vi "Init notes.vi"(11 "?":T1={"Tytuły"=[], "Folder"=path "", "Data/tytul"=[], "Ostatni index"=-10, "Title"="", "Note"=""}) -> (3 "?":T1={"Tytuły"=[], "Folder"=path "", "Data/tytul"=[], "Ostatni index"=-10, "Title"="", "Note"=""})   [LabVIEW 2020]
uses:
  #typeDef_ProgramData.ctl
  <vilib>/regexp/Match Regular Expression.xnode
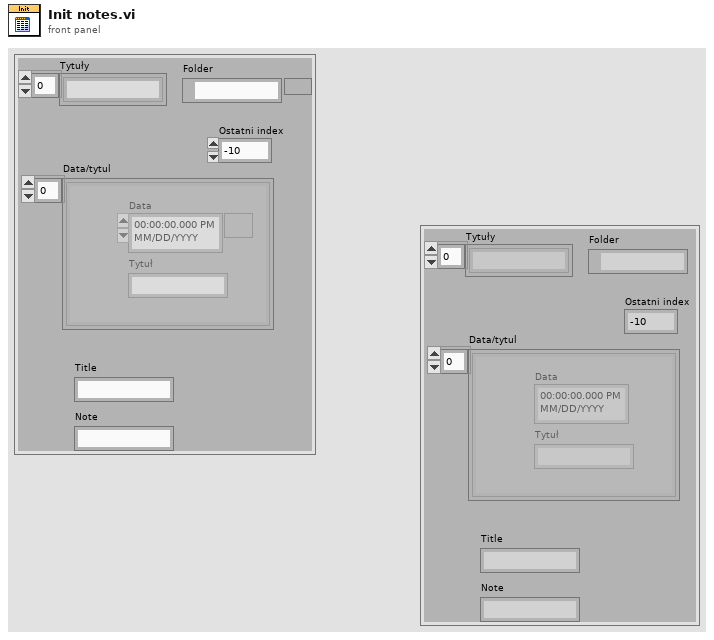
[diagram p1: front panel]
types:
  T1 = typedef "#typeDef_ProgramData.ctl" = cluster{"Tytuły":string[], "Folder":path, "Data/tytul":cluster{"Data":timestamp, "Tytuł":string}[], "Ostatni index":i32, "Title":string, "Note":string}
  T2 = cluster{"last mod":timestamp, "before match":string}
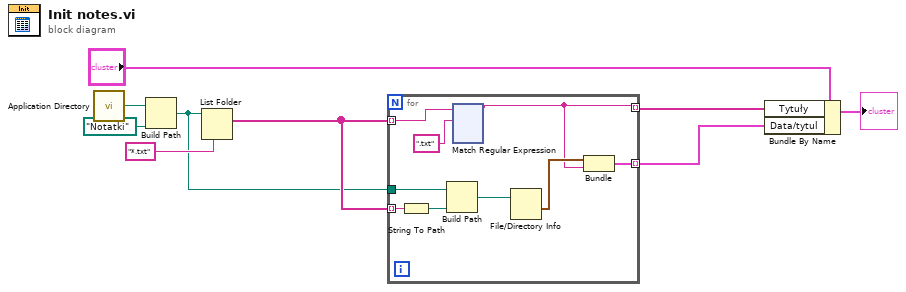
[diagram p0: block diagram]
diagram:
  n1 = call <vilib>:"Application Directory.vi"() -> ("Application Directory"=w9:path)
  n2 = Build Path(base path=w9, name or relative path=path "Notatki") -> (appended path=w3:path)
  n3 = List Folder(path=w3, pattern="*.txt") -> (filenames=w4:string[])  [unwired: 2 in, 3 out]
  n4 = for {
    tunnel: w4 -> [w17] mode=indexing
    tunnel: [w10] -> w2 mode=indexing
    tunnel: w4 -> [w15] mode=indexing
    tunnel: w3 -> [w14]
    tunnel: [w12] -> w1 mode=indexing
    n5 = String To Path(string=w15) -> (path=w13:path)
    n6 = Build Path(base path=w14, name or relative path=w13) -> (appended path=w16:path)
    n7 = xnode "Match Regular Expression"("input string"=w17, "regular expression"=".txt") -> ("before match"=w10:string)  [unwired: 4 in, 4 out]
    n8 = File/Directory Info(path=w16) -> (last mod=w11:timestamp)  [unwired: 1 in, 6 out]
    n9 = Bundle("last mod"=w11, "before match"=w10) -> (w12:T2)  [unwired: 1 in]
  }
  n10 = Bundle By Name(cluster="?", "Tytuły"=w2, "Data/tytul"=w1) -> (→"?":T1)
